vi "MultiPass - Example-Callback-VI.vi"(7 "Method":enum16{"init", "run", "end"}(ring), 8 "error in (no error)":errorcluster, 10 "Pass":i32, 11 "Line":i32) -> (0 "error out":errorcluster)   [LabVIEW 2021]
doc: "Example Multipass scanning callback VI. Increases the bias voltage for each pass.\n\n- Nanonis Programming Interface -"
uses:
  Nanonis Prog Interface.lvlib
panel:
  in  "Bias increment (V)":sgl=0.10000002 format="%#_6p"
  # "Example Callback VI for multipass scanning\nThis VI will increment the bias voltage for each pass and reset it at a new line.\n\nWorking principle of callback VIs:\nThe callback VI is called at the beginning of each scan line/pass. The line and pass numbers (both 0 based) are provided as inputs for the VI.\nThe line only increases once all passes have been finished. E.g. when doing a scan with N lines and 2 passes it will count as follows (line,pass):\n(0,0), (0,1), (0,2), (0,3), (1,0), (1,1), ..., (N-1,2), (N-1,3). \n\nEven pass numbers are forward lines, odd pass numbers are backward lines.\nThe Init method is called right after pressing the scan start buttons, and the End method is called when stopping the scan or when right after the scan finishes."
  # "Callback VI connectors"
  # "Custom controls"
  # "Don't use these on the VI connector!"
  # "Don't change the VI connector! Callback VIs must use the 4-2-2-4 connector pattern with these controls at the correct connectors to work!"
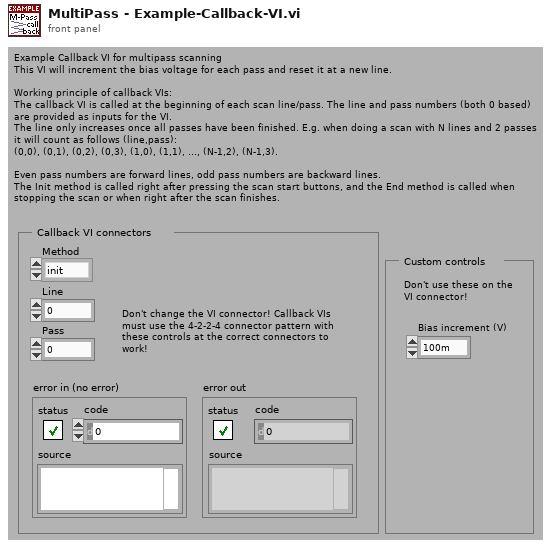
[diagram p1: front panel]
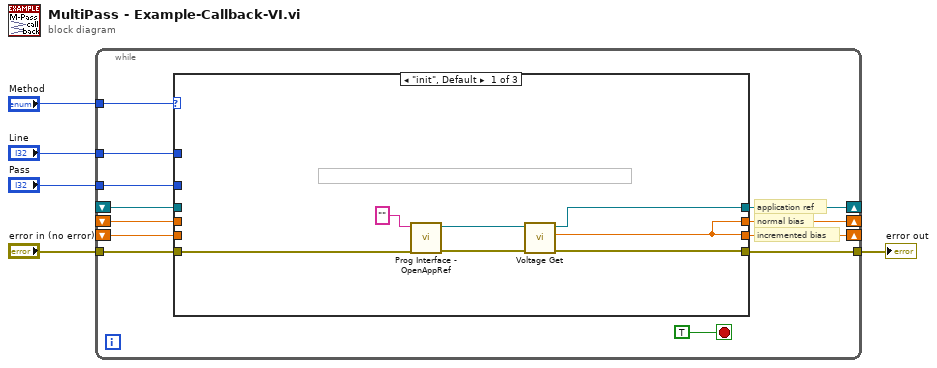
[diagram p0: block diagram]
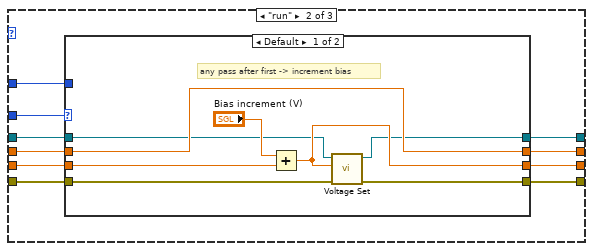
[diagram p2: hidden frame]
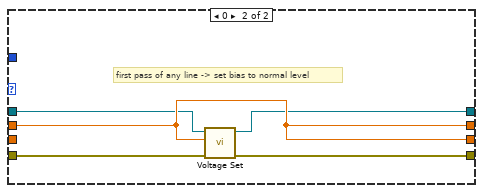
[diagram p3: hidden frame]
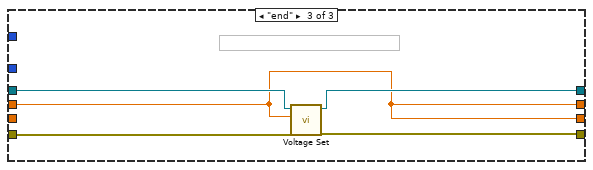
[diagram p4: hidden frame]
diagram:
  n1 = while {
    tunnel: "Pass" -> [w17]
    tunnel: "Line" -> [w16]
    shift-right: [w15] -> _
    shift-left: _ -> [w14]
    tunnel: "error in (no error)" -> [w12]
    tunnel: [w13] -> w3
    shift-right: [w10] -> _
    shift-left: _ -> [w9]
    shift-right: [w8] -> _
    shift-left: _ -> [w7]
    tunnel: "Method" -> [w6]
    stop <- TRUE stop-if-true
    # "application ref"
    # "incremented bias"
    # "normal bias"
    n2 = case shown="\"init\", Default" w6 {
      tunnel: w17 -> [_ w34 _]
      tunnel: w16 -> [_ w33 _]
      tunnel: [w20 w32 w48] -> w15
      tunnel: w14 -> [_ w31 _]
      tunnel: [w21 w30 w51] -> w13
      tunnel: w12 -> [w23 w29 w52]
      tunnel: [w20 w28 w48] -> w10
      tunnel: w9 -> [_ w27 w48]
      tunnel: [w18 w26 w49] -> w8
      tunnel: w7 -> [_ w25 w50]
      frame "init", Default {
        n3 = call <userlib>:"Prog Interface - OpenAppRef.vi"("Error in (no error)"=w23, "Machine name (local machine IP)"="") -> ("Error out"=w22:errorcluster, "Application reference"=w19:refnum<vi>)  [unwired: 4 in]
        n4 = call <userlib>:"Voltage Get.vi"("error in (no error)"=w22, "Application ref in"=w19) -> ("error out"=w21:errorcluster, "Bias (V)"=w20:sgl, "Application ref out"=w18:refnum<vi>)  [unwired: 7 in]
      }
      frame "run" {
        n5 = case shown="Default" w34 {
          tunnel: w33 -> [_ _]
          tunnel: [w38 w45] -> w32
          tunnel: w31 -> [w42 _]
          tunnel: [w39 w46] -> w30
          tunnel: w29 -> [w40 w47]
          tunnel: [w37 w45] -> w28
          tunnel: w27 -> [w37 w45]
          tunnel: [w35 w44] -> w26
          tunnel: w25 -> [w36 w43]
          frame Default {
            # "any pass after first -> increment bias"
            n6 = Add(x="Bias increment (V)", y=w42) -> (x+y=w38:sgl)
            n7 = call <userlib>:"Voltage Set.vi"("Error in (no error)"=w40, "Bias (V)"=w38, "Application ref in"=w36) -> ("Error out"=w39:errorcluster, "Application ref out"=w35:refnum<vi>)  [unwired: 7 in]
          }
          frame 0 {
            # "first pass of any line -> set bias to normal level"
            n8 = call <userlib>:"Voltage Set.vi"("Error in (no error)"=w47, "Bias (V)"=w45, "Application ref in"=w43) -> ("Error out"=w46:errorcluster, "Application ref out"=w44:refnum<vi>)  [unwired: 7 in]
          }
        }
      }
      frame "end" {
        n9 = call <userlib>:"Voltage Set.vi"("Error in (no error)"=w52, "Bias (V)"=w48, "Application ref in"=w50) -> ("Error out"=w51:errorcluster, "Application ref out"=w49:refnum<vi>)  [unwired: 7 in]
      }
    }
  }
  "error out" <- w3
